vi "Waveform.Get Subset.vi"(9 "Len":i32, 10 "Pos":i32, 11 "Data":waveform(dbl)[](array[waveform])) -> (1 "End":bool, 2 "Next Pos":i32, 3 "Data Out":waveform(dbl)[](array[waveform]))   [LabVIEW 2018]
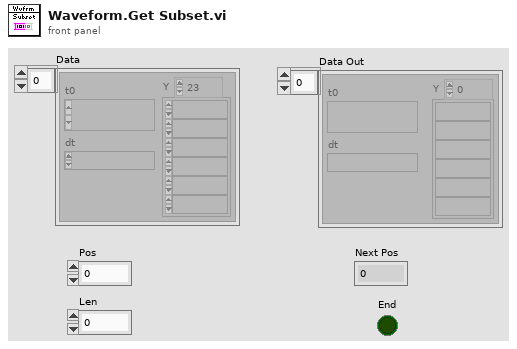
[diagram p1: front panel]
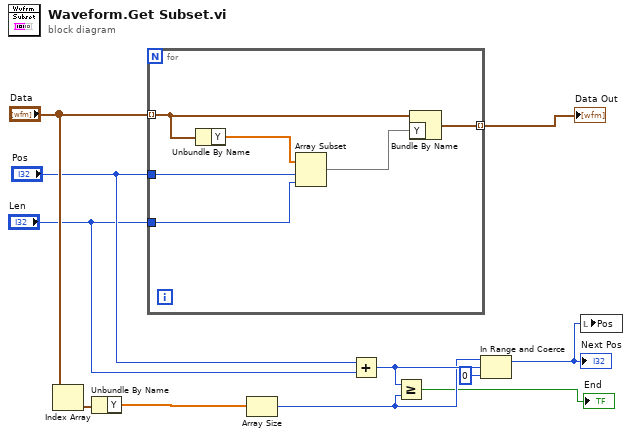
[diagram p0: block diagram]
diagram:
  n1 = Index Array(array="Data") -> (element=w9:waveform(dbl))  [unwired: 1 in]
  n2 = Unbundle By Name(w9) -> ("Y"=w8:dbl[])
  n3 = for {
    tunnel: "Data" -> [w17] mode=indexing
    tunnel: "Pos" -> [w14]
    tunnel: "Len" -> [w12]
    tunnel: [w15] -> w11 mode=indexing
    n4 = Unbundle By Name(w17) -> ("Y"=w13:dbl[])
    n5 = Array Subset(array=w13, index=w14, length=w12) -> (w16:dbl[])
    n6 = Bundle By Name(cluster=w17, "Y"=w16) -> (w15:waveform(dbl))
  }
  "Data Out" <- w11
  n7 = Array Size(array=w8) -> (size(s)=w4:i32)
  n8 = Add(x="Pos", y="Len") -> (x+y=w5:i32)
  n9 = Greater Or Equal?(x=w5, y=w4) -> (x >= y?=→"End":bool)
  n10 = In Range and Coerce(upper limit=w4, x=w5, lower limit=0) -> (coerced(x)=w1:i32)  [unwired: 1 out]
  "Next Pos" <- w1
  n11 = local write "Pos"(w1) -> ()
